vi "SendPWMProtocol.vi"(7 "Send":bool, 9 "Initialize":bool, 10 "old":T1, 11 "new":T1) -> ()   [LabVIEW 2019]
uses:
  PWM proto.ctl
  PWM data proto.ctl
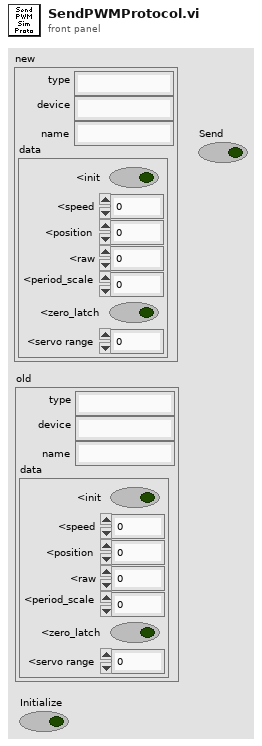
[diagram p1: front panel]
types:
  T1 = typedef "PWM proto.ctl" = cluster{"type":string, "device":string, "name":string, "data":T2}
  T2 = typedef "PWM data proto.ctl" = cluster{"<init":bool, "<speed":dbl, "<position":dbl, "<raw":dbl, "<period_scale":dbl, "<zero_latch":bool, "<servo range":dbl}
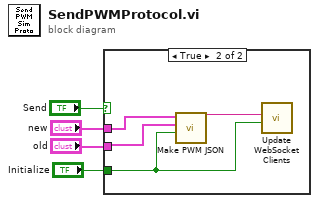
[diagram p0: block diagram]
diagram:
  n1 = case shown="True" "Send" {
    tunnel: "new" -> [_ w7]
    tunnel: "old" -> [_ w6]
    tunnel: "Initialize" -> [_ w5]
    frame False {
    }
    frame True {
      n2 = call "Make PWM JSON.vi"("Force"=w5, "PWM prev"=w6, "PWM new"=w7) -> ("delta JSON"=w8:string)  [unwired: 8 in]
      n3 = call "Update WebSocket Clients.vi"("Initialize"=w5, "delta JSON"=w8) -> ()  [unwired: 10 in]
    }
  }
